vi "TempSimulation SubVI.vi"(0 "Stopped Reference":refnum<vi>, 1 "Temperature Queue":refnum<queue>, 5 "Temperatures":T4, 7 "Frequency":dbl, 9 "LightCases":T1, 11 "error in (no error)":errorcluster, 12 "TemperatureData":T2) -> (3 "F0 Temp Chart":dbl(graph), 4 "F0 Gain":dbl, 6 "F1 Temp Chart":dbl(graph), 8 "F1 Gain":dbl, 10 "Kinti hõmérséklet":dbl, 15 "error out":errorcluster)   [LabVIEW 2014]
uses:
  Types/TemperatureArray.ctl
  Types/TemperatureControlData.ctl
  Types/HeatingMode.ctl
  Types/LightCases.ctl
  Types/FVGFuncts.ctl
  <vilib>/express/express arith-compare/Formula/XNode/ExpressFormulaBlockNode.xnode
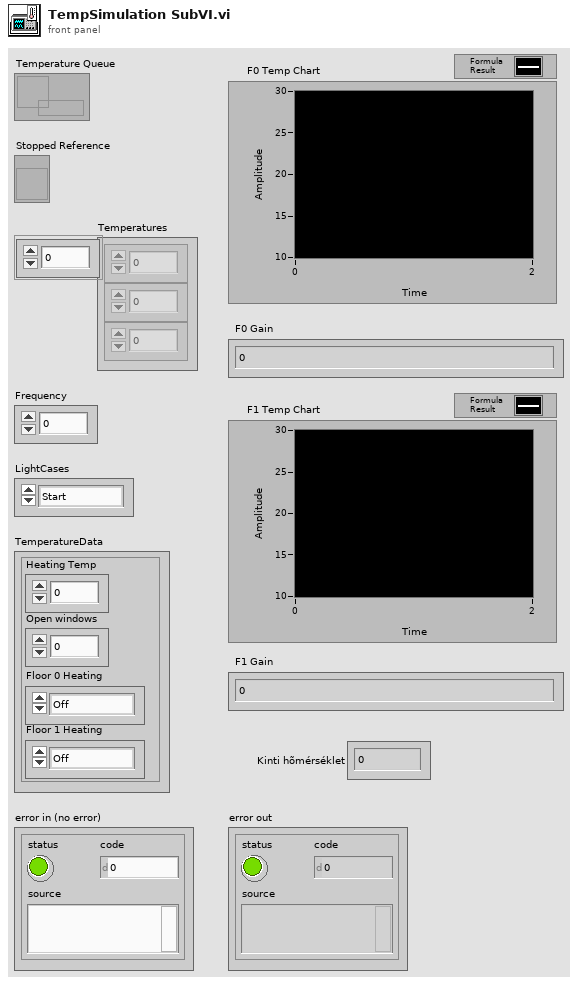
[diagram p1: front panel]
types:
  T1 = typedef "LightCases.ctl" = enum16{"Start", "Update", "Stop"}
  T2 = typedef "TemperatureControlData.ctl" = cluster{"Open windows":dbl, "Floor 0 Heating":T3, "Floor 1 Heating":T3, "Heating Temp":dbl}
  T3 = typedef "HeatingMode.ctl" = enum16{"Off", "Heating", "Cooling"}
  T4 = typedef "TemperatureArray.ctl" = dbl[]
  T5 = typedef "FVGFuncts.ctl" = enum16{"Init", "Set Data", "Get Data"}
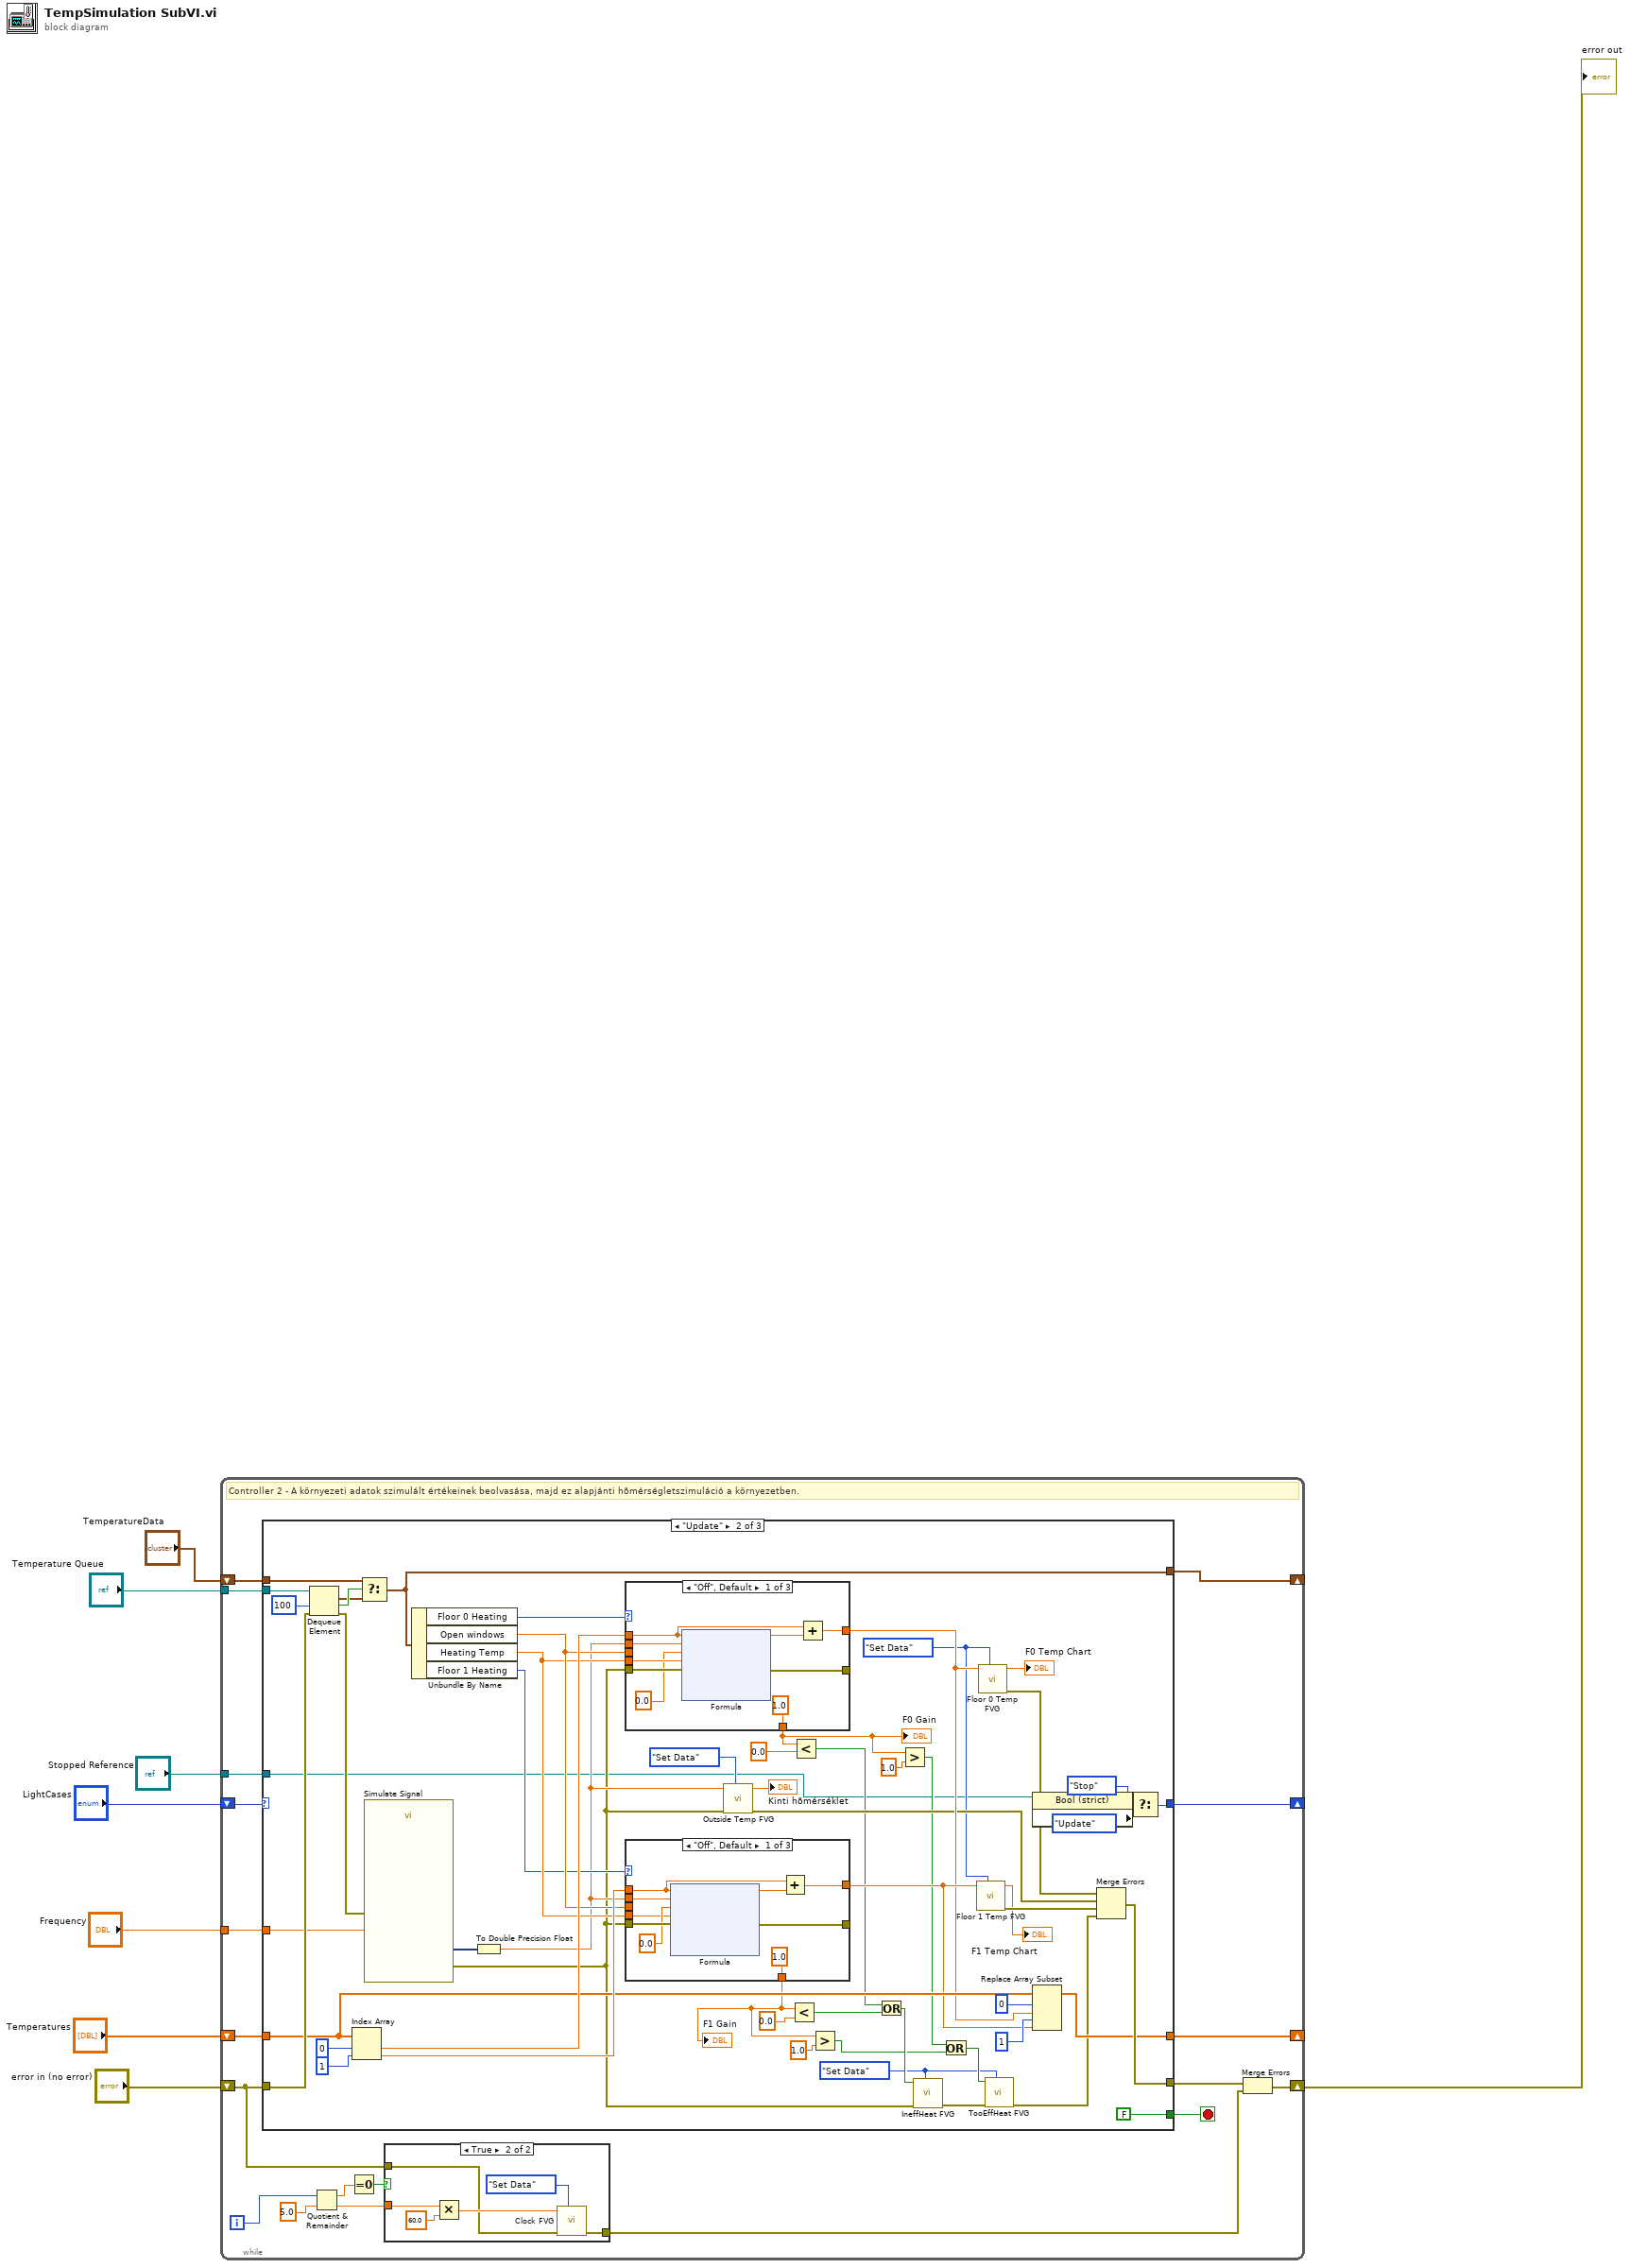
[diagram p0: block diagram]
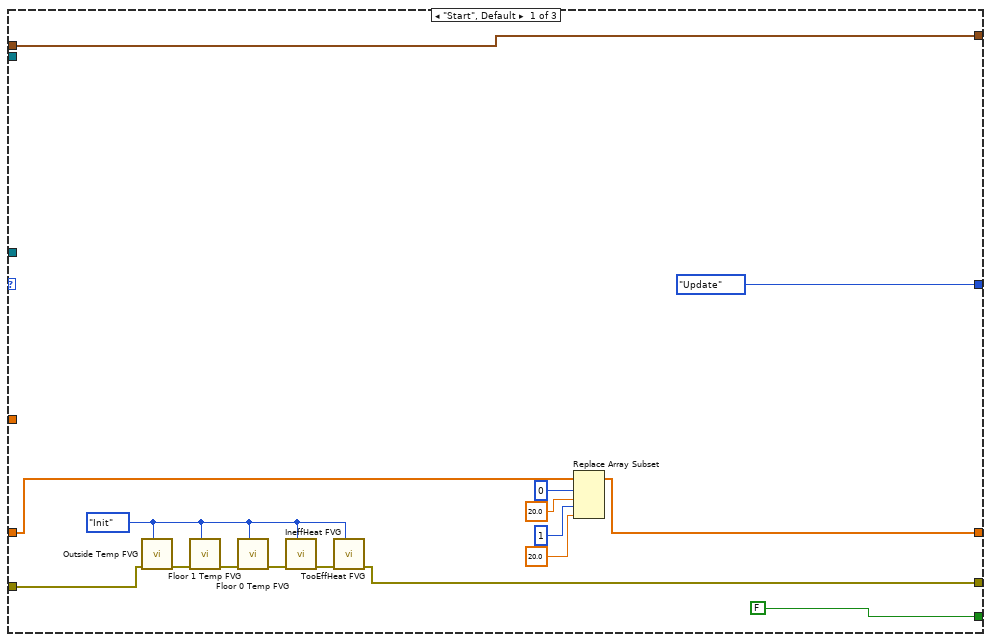
[diagram p2: hidden frame]
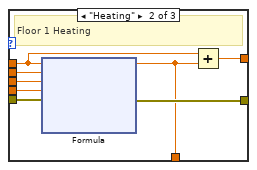
[diagram p3: hidden frame]
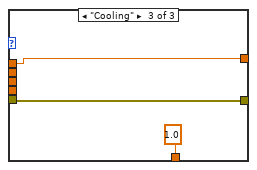
[diagram p4: hidden frame]
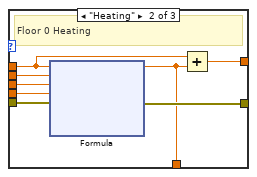
[diagram p5: hidden frame]
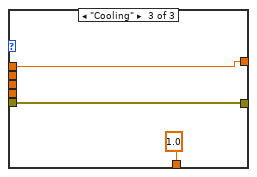
[diagram p6: hidden frame]
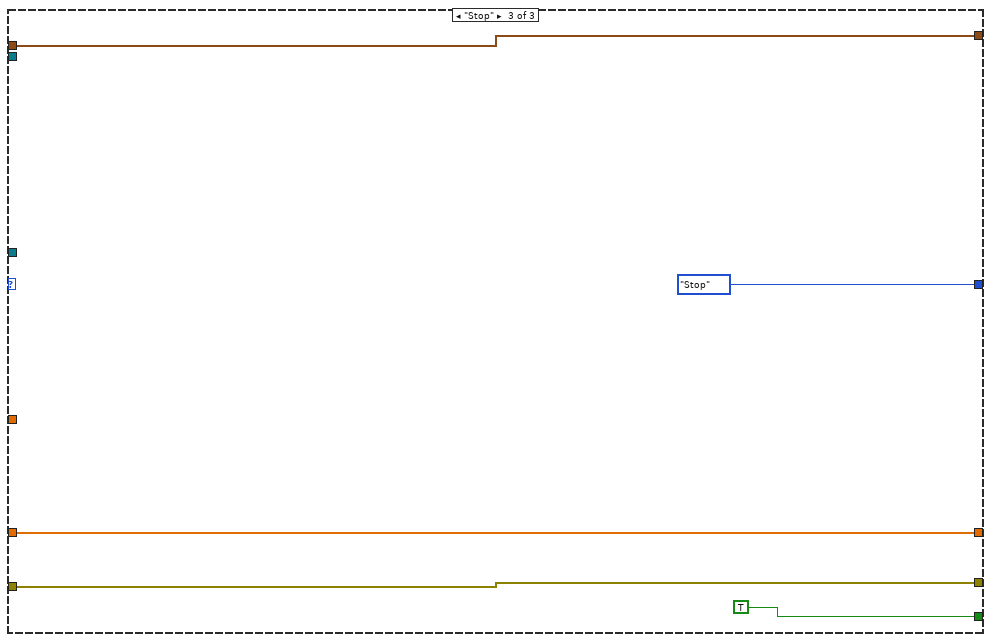
[diagram p7: hidden frame]
diagram:
  n1 = while {
    tunnel: "Temperature Queue" -> [w27]
    shift-right: [w12] -> w6
    shift-left: "error in (no error)" -> [w13]
    shift-right: [w24] -> _
    shift-left: "LightCases" -> [w25]
    shift-right: [w22] -> _
    shift-left: "TemperatureData" -> [w23]
    tunnel: "Frequency" -> [w21]
    shift-right: [w19] -> _
    shift-left: "Temperatures" -> [w20]
    tunnel: "Stopped Reference" -> [w9]
    i -> [w18]
    stop <- w26 stop-if-true
    # "Controller 2 - A környezeti adatok szimulált értékeinek beolvasása, majd ez alapjánti hõmérségletszimuláció a környezetben."
    n2 = case shown="\"Update\"" w25 {
      tunnel: w27 -> [_ w98 _]
      tunnel: w13 -> [w29 w97 w197]
      tunnel: [FALSE FALSE TRUE] -> w26
      tunnel: [LightCases."Update" w88 LightCases."Stop"] -> w24
      tunnel: w23 -> [w41 w95 w200]
      tunnel: [w41 w76 w200] -> w22
      tunnel: [w28 w86 w197] -> w11
      tunnel: w21 -> [_ w87 _]
      tunnel: w20 -> [w40 w78 w196]
      tunnel: [w35 w77 w196] -> w19
      tunnel: w9 -> [_ w44 _]
      frame "Start", Default {
        w30 = FVGFuncts."Init" ("Enum")
        n3 = call "Outside Temp FVG.vi"("Mode"=w30, "Error In"=w29) -> ("Error Out"=w33:errorcluster)  [unwired: 8 in, 1 out]
        n4 = call "Floor 1 Temp FVG.vi"("Mode"=w30, "Error In"=w33) -> ("Error Out"=w34:errorcluster)  [unwired: 8 in, 1 out]
        n5 = call "Floor 0 Temp FVG.vi"("Mode"=w30, "Error In"=w34) -> ("Error Out"=w32:errorcluster)  [unwired: 8 in, 1 out]
        n6 = call "IneffHeat FVG.vi"("Mode"=w30, "Error In"=w32) -> ("Error Out"=w31:errorcluster)  [unwired: 8 in, 1 out]
        n7 = call "TooEffHeat FVG.vi"("Mode"=w30, "Error In"=w31) -> ("Error Out"=w28:errorcluster)  [unwired: 8 in, 1 out]
        n8 = Replace Array Subset(array=w40, new element #1=20.0 ("new element/subarray"), index #1=0 ("index"), new element #2=20.0 ("new element/subarray"), index #2=1 ("index")) -> (w35:T4)
      }
      frame "Update" {
        w45 = FVGFuncts."Set Data" ("Mode")
        w50 = FVGFuncts."Set Data" ("Enum")
        n9 = Dequeue Element(queue=w98, timeout in ms (-1)=100, error in (no error)=w97) -> (element=w93:T2, timed out?=w94:bool, error out=w92:errorcluster)  [unwired: 1 out]
        n10 = Index Array(array=w78, index #1=0 ("index"), index #2=1 ("index")) -> (element #1=w81:dbl, element #2=w80:dbl)
        n11 = Select(t=w95, s=w94, f=w93) -> (s? t:f=w76:T2)
        n12 = call "Simulate Signal"("Frequency"=w87, "error in (no error)"=w92) -> ("Outside temperature"=w79:dynamicdata, "error out"=w57:errorcluster)  [unwired: 12 in]
        n13 = Unbundle By Name(w76) -> ("Floor 0 Heating"=w75:T3, "Open windows"=w74:dbl, "Heating Temp"=w73:dbl, "Floor 1 Heating"=w72:T3)
        n14 = To Double Precision Float(number=w79) -> (double precision float=w65:dbl)
        n15 = case shown="\"Off\", Default" w75 {
          tunnel: [w152 w178 w195] -> _
          tunnel: w57 -> [w156 w177 w195]
          tunnel: w81 -> [w148 w172 w194]
          tunnel: w65 -> [w153 w176 _]
          tunnel: w74 -> [_ w175 _]
          tunnel: w73 -> [w155 w174 _]
          tunnel: [w150 w173 w194] -> w69
          tunnel: [1.0 ("Result") w171 1.0 ("Result")] -> w52
          frame "Off", Default {
            n16 = xnode "Formula"("T_szoba"=w148, "T_kint"=w153, "H_on"=0.0, "T_h"=w155, "error in (no error)"=w156) -> ("Result"=w149:dbl, "error out"=w152:errorcluster)
            n17 = Add(x=w148, y=w149) -> (x+y=w150:dbl)
          }
          frame "Heating" {
            # "Floor 0 Heating"
            n18 = xnode "Formula"("T_szoba"=w172, "T_kint"=w176, "H_on"=w175, "T_h"=w174, "error in (no error)"=w177) -> ("Result"=w171:dbl, "error out"=w178:errorcluster)
            n19 = Add(x=w172, y=w171) -> (x+y=w173:dbl)
          }
          frame "Cooling" {
          }
        }
        "F0 Gain" <- w52
        n20 = case shown="\"Off\", Default" w72 {
          tunnel: [w104 w130 w146] -> _
          tunnel: w57 -> [w108 w129 w146]
          tunnel: w80 -> [w102 w125 w147]
          tunnel: w65 -> [w105 w128 _]
          tunnel: [w100 w124 w147] -> w71
          tunnel: w74 -> [_ w127 _]
          tunnel: w73 -> [w106 w126 _]
          tunnel: [1.0 ("Result") w123 1.0 ("Result")] -> w47
          frame "Off", Default {
            n21 = xnode "Formula"("T_szoba"=w102, "T_kint"=w105, "H_on"=0.0, "T_h"=w106, "error in (no error)"=w108) -> ("Result"=w101:dbl, "error out"=w104:errorcluster)
            n22 = Add(x=w102, y=w101) -> (x+y=w100:dbl)
          }
          frame "Heating" {
            # "Floor 1 Heating"
            n23 = xnode "Formula"("T_szoba"=w125, "T_kint"=w128, "H_on"=w127, "T_h"=w126, "error in (no error)"=w129) -> ("Result"=w123:dbl, "error out"=w130:errorcluster)
            n24 = Add(x=w125, y=w123) -> (x+y=w124:dbl)
          }
          frame "Cooling" {
          }
        }
        "F1 Gain" <- w47
        n25 = call "Outside Temp FVG.vi"("Mode"=FVGFuncts."Set Data" ("Enum"), "Error In"=w57, "Data In"=w65) -> ("Error Out"=w66:errorcluster, "Data Out"=→"Kinti hõmérséklet":dbl)  [unwired: 7 in]
        n26 = Less?(x=w47, y=0.0) -> (x < y?=w60:bool)
        n27 = Less?(x=w52, y=0.0) -> (x < y?=w59:bool)
        n28 = Greater?(x=w47, y=1.0) -> (0:w46:bool)
        n29 = Or(x=w59, y=w60) -> (x .or. y?=w56:bool)
        n30 = Greater?(x=w52, y=1.0) -> (0:w49:bool)
        n31 = call "IneffHeat FVG.vi"("Mode"=w45, "Error In"=w57, "Data In"=w56) -> ("Error Out"=w54:errorcluster)  [unwired: 7 in, 1 out]
        n32 = Or(x=w49, y=w46) -> (x .or. y?=w53:bool)
        n33 = call "Floor 1 Temp FVG.vi"("Mode"=w50, "Data In"=w71) -> ("Error Out"=w70:errorcluster, "Data Out"=→"F1 Temp Chart":dbl)  [unwired: 8 in]
        n34 = call "Floor 0 Temp FVG.vi"("Mode"=w50, "Data In"=w69) -> ("Error Out"=w67:errorcluster, "Data Out"=→"F0 Temp Chart":dbl)  [unwired: 8 in]
        n35 = call "TooEffHeat FVG.vi"("Mode"=w45, "Error In"=w54, "Data In"=w53) -> ("Error Out"=w55:errorcluster)  [unwired: 7 in, 1 out]
        n36 = property class="Bool (strict)"(reference=w44) -> ("Value"=w90:bool)  [unwired: 1 in, 2 out]
        n37 = Replace Array Subset(array=w78, new element #1=w69, index #1=0 ("index"), new element #2=w71, index #2=1 ("index")) -> (w77:T4)
        n38 = Merge Errors(w67, w66, w70, w55) -> (w86:errorcluster)
        n39 = Select(t=LightCases."Stop", s=w90, f=LightCases."Update") -> (s? t:f=w88:T1)
      }
      frame "Stop" {
      }
    }
    n40 = Quotient & Remainder(x=w18, y=5.0) -> (x-y*floor(x/y)=w14:dbl, floor(x/y)=w16:dbl)
    n41 = Equal To 0?(x=w14) -> (x = 0?=w15:bool)
    n42 = case shown="True" w15 {
      tunnel: w16 -> [_ w206]
      tunnel: w13 -> [w201 w203]
      tunnel: [w201 w202] -> w10
      frame False {
      }
      frame True {
        n43 = Multiply(x=w206, y=60.0) -> (x*y=w204:dbl)
        n44 = call "Clock FVG.vi"("Mode"=FVGFuncts."Set Data", "Error In"=w203, "Data In"=w204) -> ("Error Out"=w202:errorcluster)  [unwired: 7 in, 1 out]
      }
    }
    n45 = Merge Errors(w11, w10) -> (w12:errorcluster)
  }
  "error out" <- w6
